vi "LinearQuadraticRegulator_New_ELMS.vi"(5 "States":i32, 6 "dt_Seconds":dbl=0.02, 7 "Inputs":i32, 8 "Relms":T2, 9 "Qelms":T2, 10 "B":T2, 11 "A":T2) -> (0 "Error":bool, 3 "LinearQuadraticRegulator":T1)   [LabVIEW 2019, in "Trajectory_Library.lvlib"]
doc: "Creates a new LINEAR SYSTEM data cluster with the specified values. \n\n\nInputs: \n - XXX -- XXX.\n\nOutputs:\n - XXX -- XXX."
uses:
  Trajectory_Library.lvlib
  <vilib>/Analysis/Matrix/Datatypes/RealMatrix.ctl
  LINEAR_QUADRATIC_REGULATOR.ctl
  MatBuilder_Create.vi
  <vilib>/Analysis/Matrix/NI_Matrix.lvlib
panel:
  # "<States,States>"
  # "<States,Inputs>"
  # "<States,1>"
  # "<Inputs,1>"
  # "Ref State <States,1>"
  # "Comp and capped \noutput <Inputs,1>"
  # "Controller gain\n<Inputs,States>"
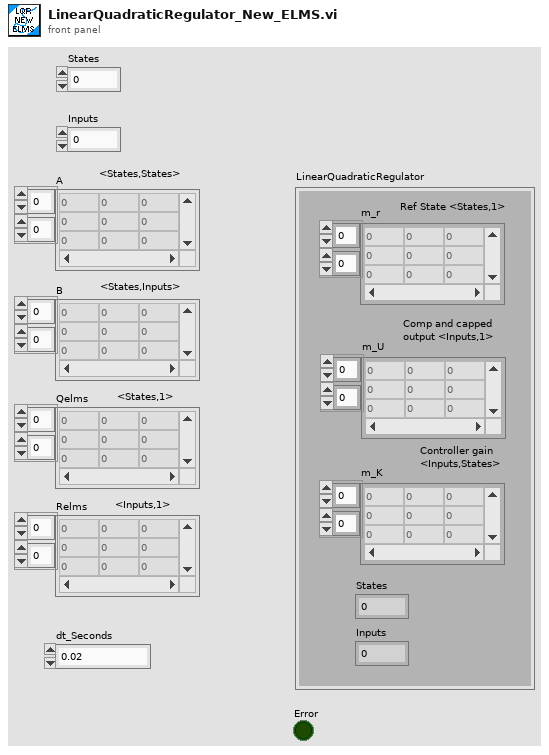
[diagram p1: front panel]
types:
  T1 = typedef "Trajectory_Library.lvlib/LINEAR_QUADRATIC_REGULATOR.ctl" = cluster{"m_r":T2, "m_U":T2, "m_K":T2, "States":i32, "Inputs":i32}
  T2 = typedef "NI_Matrix.lvlib/RealMatrix.ctl" = dbl[][]
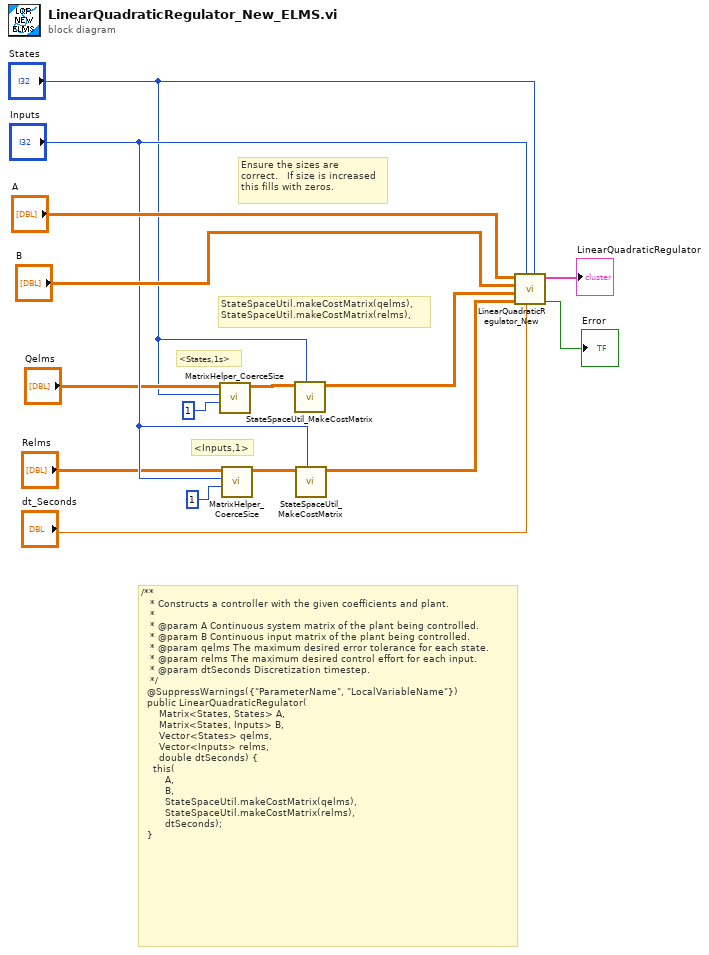
[diagram p0: block diagram]
diagram:
  # "StateSpaceUtil.makeCostMatrix(qelms),\nStateSpaceUtil.makeCostMatrix(relms),"
  # "<Inputs,1>"
  # "<States,1s>"
  # "Ensure the sizes are\ncorrect.   If size is increased \nthis fills with zeros."
  # "/**\n   * Constructs a controller with the given coefficients and plant.\n   *\n   * @param A Continuous system matrix of the plant being controlled.\n   * @param B Continuous input matrix of the plant being controlled.\n   * @param qelms The maximum desired error tolerance for each state.\n   * @param relms The maximum desired control effort for each input.\n   * @param dtSeconds Discretization timestep.\n   */\n  @SuppressWarnings({\"ParameterName\", \"LocalVariableName\"})\n  public LinearQuadraticRegulator(\n      Matrix<States, States> A,\n      Matrix<States, Inputs> B,\n      Vector<States> qelms,\n      Vector<Inputs> relms,\n      double dtSeconds) {\n    this(\n        A,\n        B,\n        StateSpaceUtil.makeCostMatrix(qelms),\n        StateSpaceUtil.makeCostMatrix(relms),\n        dtSeconds);\n  }"
  n1 = call "MatrixHelper_CoerceSize.vi"("Columns"=1 ("number of columns"), "Rows"="States", "input matrix"="Qelms") -> ("output matrix"=w4:T2)  [unwired: 8 in]
  n2 = call "MatrixHelper_CoerceSize.vi"("Columns"=1 ("number of columns"), "Rows"="Inputs", "input matrix"="Relms") -> ("output matrix"=w5:T2)  [unwired: 8 in]
  n3 = call "StateSpaceUtil_MakeCostMatrix.vi"("States"="States", "Costs"=w4) -> ("Costs Matrix"=w12:T2)  [unwired: 9 in]
  n4 = call "StateSpaceUtil_MakeCostMatrix.vi"("States"="Inputs", "Costs"=w5) -> ("Costs Matrix"=w11:T2)  [unwired: 9 in]
  n5 = call "LinearQuadraticRegulator_New.vi"("States"="States", "dt_Seconds"="dt_Seconds", "Inputs"="Inputs", "R"=w11, "Q"=w12, "B"="B", "A"="A") -> ("Error"=→"Error":bool, "LinearQuadraticRegulator"=→"LinearQuadraticRegulator":T1)  [unwired: 3 in]
